vi "Calculate Speed.vi"(1 "dimension":dbl, 2 "rotational":dbl, 3 "translational":dbl) -> (0 "speed":dbl)   [LabVIEW 2014]
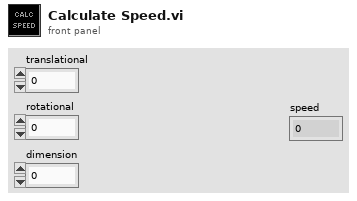
[diagram p1: front panel]
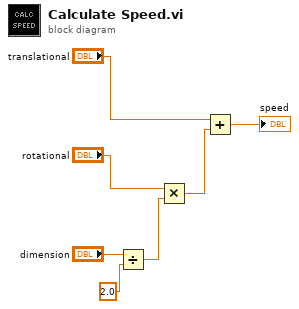
[diagram p0: block diagram]
diagram:
  n1 = Divide(x="dimension", y=2.0) -> (x/y=w5:dbl)
  n2 = Multiply(x="rotational", y=w5) -> (x*y=w2:dbl)
  n3 = Add(x="translational", y=w2) -> (x+y=→"speed":dbl)
